vi "_NO_NTJ_OldVer_FlushSingle.vi"(8 "error in (no error)":errorcluster, 11 "Entry Name":string) -> (0 "error out":errorcluster)   [LabVIEW 2019]
uses:
  <vilib>/Rock Robotics/Network Tables/Create Actual Table Name.vi
  From_NTJ/NTJ_Convert NT Boolean to LV String.vi
  From_NTJ/NTJ_Convert String to NT Boolean Array Buffer.vi
  From_NTJ/NTJ_Convert String to NT Numeric Array Buffer.vi
  From_NTJ/NTJ_Convert String to NT String Array Buffer.vi
  <vilib>/Rock Robotics/Network Tables/Convert NT Types.vi
  From_NTJ/NTJ_Build NT Field ID Buffer.vi
  <vilib>/Utility/error.llb/Clear Errors.vi
  <vilib>/Rock Robotics/Network Tables/NT Globals.vi
  <vilib>/Rock Robotics/Network Tables/Table Manager.vi
  <vilib>/Rock Robotics/Network Tables/Log Issues.vi
  From_NTJ/NTJ_Convert String to NT String Buffer.vi
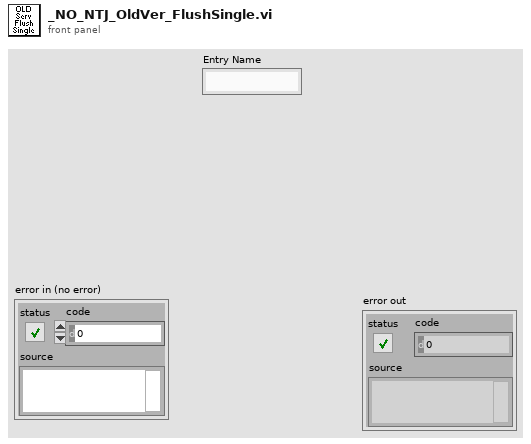
[diagram p1: front panel]
types:
  T1 = typedef "Field ID.ctl" = i32
  T2 = enum16{"Add Cnx", "Remove Cnx", "Retrieve List", "Cnx Inited"}
  T3 = enum16{"Update Field", "Read Field", "Assign Field", "Remove All", "Set Persistence", "Clear Persistence"}
  T4 = typedef "Field Data.ctl" = cluster{"Dbl":dbl, "String":string, "Type":T5, "Boolean":bool, "Sequence #":T6, "Flags":u8}
  T5 = typedef "Field Type.ctl" = enum8{"Invalid", "Bool", "Numeric", "String", "Raw", "Boolean Array", "Numeric Array", "String Array", "RPC"}
  T6 = typedef "Sequence.ctl" = u16
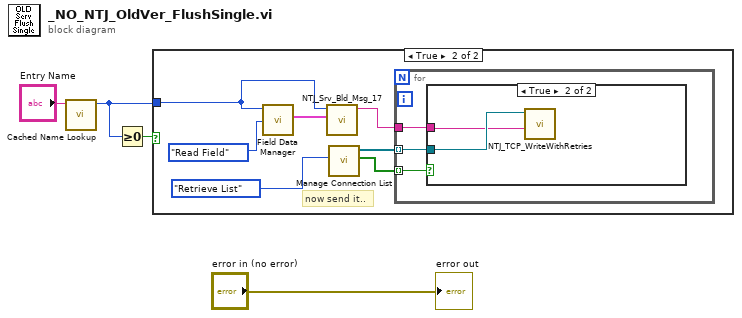
[diagram p0: block diagram]
diagram:
  n1 = call <vilib>:"Cached Name Lookup.vi"("Name"="Entry Name") -> ("Entry ID"=w4:T1)  [unwired: 8 in, 2 out]
  n2 = Greater Or Equal To 0?(x=w4) -> (x >= 0?=w3:bool)
  n3 = case shown="True" w3 {
    tunnel: w4 -> [_ w10]
    frame False {
    }
    frame True {
      # "now send it.."
      n4 = call <vilib>:"Field Data Manager.vi"("Operation"=T3."Read Field", "Field ID"=w10) -> ("Field Value Out"=w9:T4)  [unwired: 8 in, 1 out]
      n5 = call "NTJ_Srv_Bld_Msg_17.vi"("Field Value"=w9, "Field ID"=w10) -> ("Msg Buffer"=w5:string)  [unwired: 9 in]
      n6 = call <vilib>:"Manage Connection List.vi"("Operation"=T2."Retrieve List") -> ("Inited"=w6:bool[], "Connections List"=w7:refnum<k5>[])  [unwired: 8 in, 1 out]
      n7 = for {
        tunnel: w7 -> [w13] mode=indexing
        tunnel: w6 -> [w14] mode=indexing
        tunnel: w5 -> [w12]
        n8 = case shown="True" w14 {
          tunnel: w13 -> [_ w16]
          tunnel: w12 -> [_ w15]
          frame False {
          }
          frame True {
            n9 = call "NTJ_TCP_WriteWithRetries.vi"("Msg Buffer"=w15, "TCP Network Connection in"=w16) -> ()  [unwired: 8 in, 2 out]
          }
        }
      }
    }
  }
  "error out" <- "error in (no error)"
